vi "replace tag.vi"(8 "error in":errorcluster, 10 "tag to set":refnum<class "data bus tag description.lvclass">, 11 "tag collection in":refnum<class "data bus tag collection.lvclass">) -> (0 "error out":errorcluster, 3 "tag collection out":refnum<class "data bus tag collection.lvclass">)   [LabVIEW 2013, in "data bus tag collection.lvclass"]
uses:
  data bus tag collection.lvclass
  tag/data bus tag description.lvclass
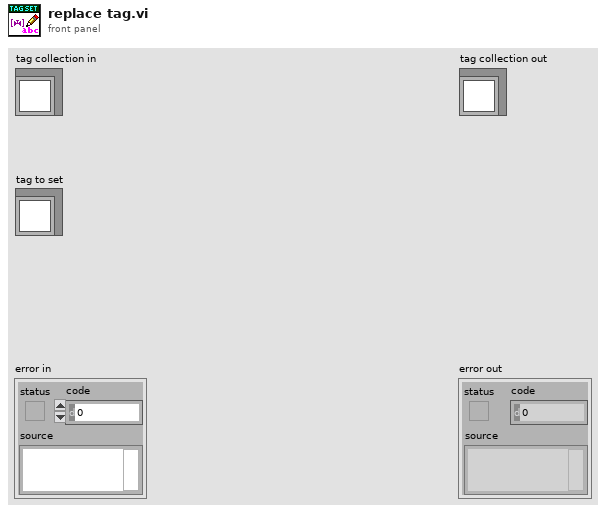
[diagram p1: front panel]
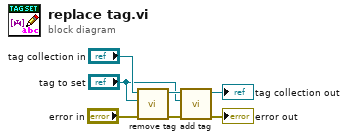
[diagram p0: block diagram]
diagram:
  n1 = call "remove tag.vi"("error in"="error in", "tag"="tag to set", "tag collection in"="tag collection in") -> ("error out"=w5:errorcluster, "tag collection out"=w4:refnum<class "data bus tag collection.lvclass">)  [unwired: 6 in, 1 out]
  n2 = call "add tag.vi"("error in"=w5, "tag"="tag to set", "tag collection in"=w4) -> ("error out"=→"error out":errorcluster, "tag collection out"=→"tag collection out":refnum<class "data bus tag collection.lvclass">)  [unwired: 7 in]
